vi "UpdateCamTestEvents.vi"(8 "error in (no error)":errorcluster, 10 "CameraTestingEvnt":T1, 11 "CameraTestingENI":refnum<class "CameraTestingENI.lvclass">) -> (0 "error out":errorcluster, 3 "CameraTestingENI":refnum<class "CameraTestingENI.lvclass">)   [LabVIEW 2020, in "CameraTestingProxy.lvlib" / "CameraTestingENI.lvclass"]
uses:
  CameraTestingENI.lvclass
  CameraTestingApp/ICameraTesting/TypeDef/Events.ctl
  Camera/ICamera/TypeDef/SnapInfo.ctl
  CameraTestingApp/ICameraTesting/TypeDef/FrameRateValReceived.ctl
  CameraTestingApp/ICameraTesting/TypeDef/ImgTypeValReceived.ctl
  CameraTestingApp/ICameraTesting/TypeDef/ResolutionValReceived.ctl
  CameraTestingApp/ICameraTesting/TypeDef/VideoOptCodesUpdated.ctl
  CameraTestingApp/ICameraTesting/TypeDef/VideoOptionsInfo.ctl
  CameraTestingApp/ICameraTesting/TypeDef/StatusUpdated.ctl
  CameraTestingApp/ICameraTesting/TypeDef/StatusRecord.ctl
  CameraTestingApp/ICameraTesting/TypeDef/VideoBufferUpdate.ctl
  CameraTestingENI.lvclass/CameraTestingENI.ctl
  <vilib>/event_ctls.llb/usereventprio.ctl
  Camera/ICamera/TypeDef/ICamera_typedef.lvlib
  CameraTestingApp/ICameraTesting/TypeDef/ICameraTesting_typedef.lvlib
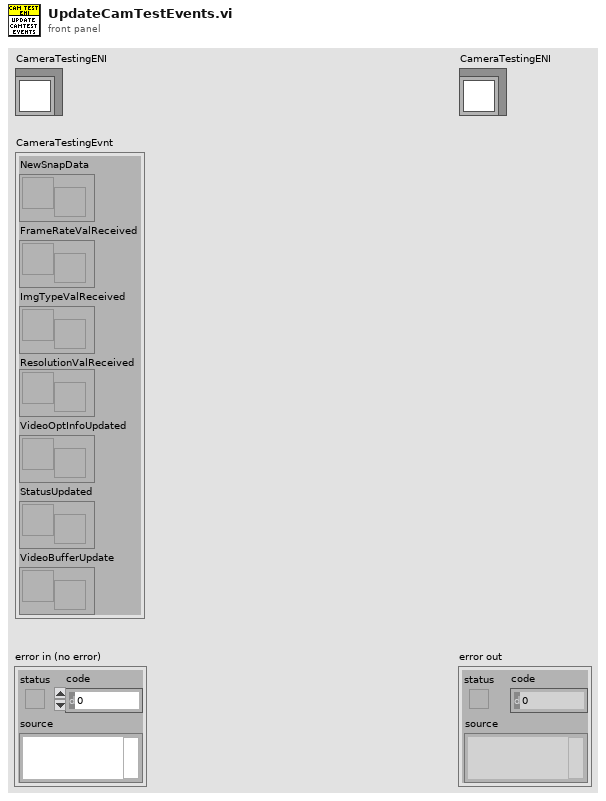
[diagram p1: front panel]
types:
  T1 = typedef "ICameraTesting_typedef.lvlib/Events.ctl" = cluster{"NewSnapData":refnum<user-event>, "FrameRateValReceived":T2, "ImgTypeValReceived":T3, "ResolutionValReceived":T4, "VideoOptInfoUpdated":T5, "StatusUpdated":T6, "VideoBufferUpdate":T7}
  T2 = typedef "ICameraTesting_typedef.lvlib/FrameRateValReceived.ctl" = refnum<user-event>
  T3 = typedef "ICameraTesting_typedef.lvlib/ImgTypeValReceived.ctl" = refnum<user-event>
  T4 = typedef "ICameraTesting_typedef.lvlib/ResolutionValReceived.ctl" = refnum<user-event>
  T5 = typedef "ICameraTesting_typedef.lvlib/VideoOptCodesUpdated.ctl" = refnum<user-event>
  T6 = typedef "ICameraTesting_typedef.lvlib/StatusUpdated.ctl" = refnum<user-event>
  T7 = typedef "ICameraTesting_typedef.lvlib/VideoBufferUpdate.ctl" = refnum<user-event>
  T8 = typedef "usereventprio.ctl" = enum32{"high priority", "normal priority"}
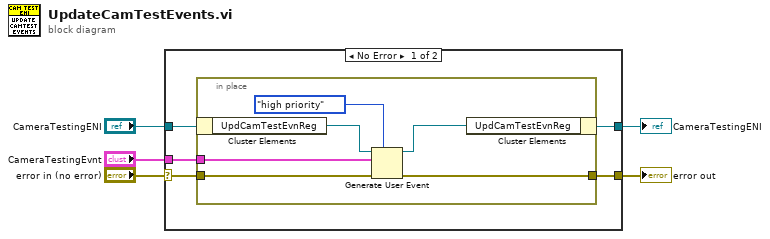
[diagram p0: block diagram]
diagram:
  n1 = case shown="No Error" "error in (no error)" {
    selector: "error in (no error)" -> [w7 w18]
    tunnel: "CameraTestingENI" -> [w10 w17]
    tunnel: "CameraTestingEvnt" -> [w9 _]
    tunnel: [w6 w18] -> w1
    tunnel: [w8 w17] -> w4
    frame No Error {
      n2 = in-place {
        in-place-border: w9 -> [w14]
        in-place-border: w7 -> [w16]
        in-place-border: [w12] -> w6
        n3 = in-place-cluster #1(w10) -> ("UpdCamTestEvnReg"=w15:refnum<user-event>)
        n4 = Generate User Event(priority (normal)=usereventprio."high priority", user event=w15, event data cluster=w14, error in=w16) -> (user event out=w13:refnum<user-event>, error out=w12:errorcluster)
        n5 = in-place-cluster #1("UpdCamTestEvnReg"=w13) -> (w8:refnum<class "CameraTestingENI.lvclass">)
      }
    }
    frame Error {
    }
  }
  "error out" <- w1
  "CameraTestingENI" <- w4
